vi "Update UI Captions.vi"(7 "Diagnostic Protocol":T1, 8 "error in (no error)":errorcluster, 10 "Cmd":T3, 11 "UI.Refs":T2) -> (0 "error out":errorcluster)   [LabVIEW 2015, in "Diagnostics Addon Shared.lvlib"]
uses:
  Diagnostics Addon Shared.lvlib
  Types/Channel Commands Enum.ctl
  Types/UI.Refs.ctl
  Types/Diagnostic Protocols.ctl
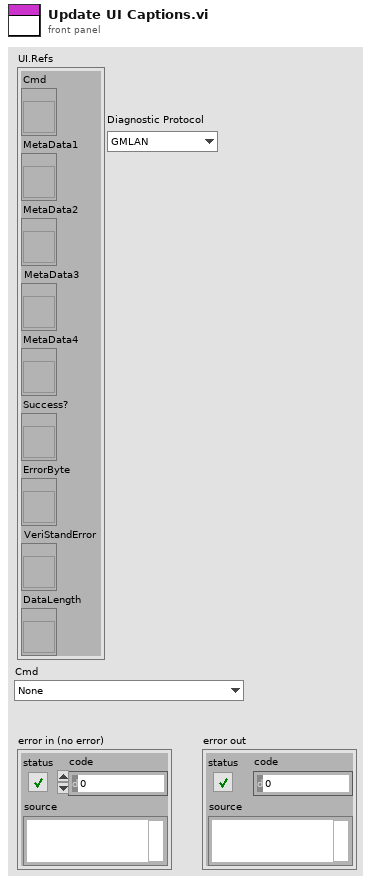
[diagram p1: front panel]
types:
  T1 = typedef "Diagnostics Addon Shared.lvlib/Diagnostic Protocols.ctl" = enum16{"GMLAN", "KWP-2000", "UDS"}
  T2 = typedef "Diagnostics Addon Shared.lvlib/UI.Refs.ctl" = cluster{"Cmd":refnum<vi>, "MetaData1":refnum<vi>, "MetaData2":refnum<vi>, "MetaData3":refnum<vi>, "MetaData4":refnum<vi>, "Success?":refnum<vi>, "ErrorByte":refnum<vi>, "VeriStandError":refnum<vi>, "DataLength":refnum<vi>}
  T3 = typedef "Diagnostics Addon Shared.lvlib/Channel Commands Enum.ctl" = enum8{"None", "EnableDiagnosticSession", "DisableDiagnosticSession", "ReadDataIdentifiers", "ReadDataIdentifier", "WriteDataIndentifier", "ReadPIDsOnDemand", "ReadPIDOnDemand", "WriteCPID", "WriteMemory", "ReadMemory", "ReadDTCs", "ClearDTCs", "ControlDTC", "ForceTesterPresent", "DisableNormalCommunication", "ReturnToNormalMode", "InputOutputControl", "StartRoutine", "RequestRoutineStatus", "StopRoutine", "ECUReset", "UnlockECU", "ClearSuccessBit", "ConfigureandStartPIDs", "StopPIDs", "StartDTCs", "EnableChangeDTCCount", "DisableChangeDTCCount", "ReadFailureRecordParameters", "PassThru Channel Based"}
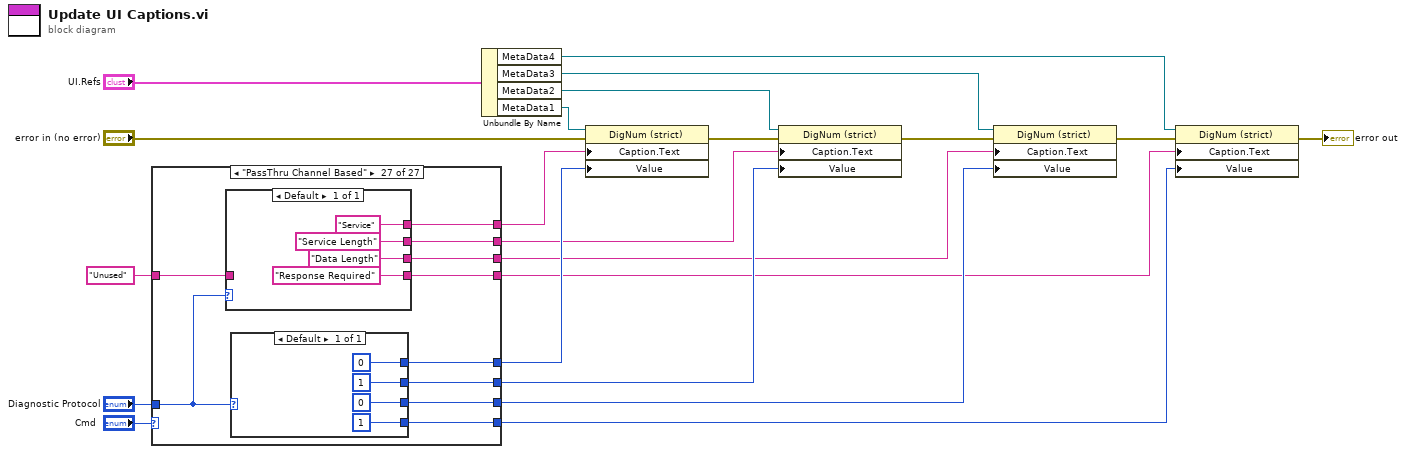
[diagram p0: block diagram]
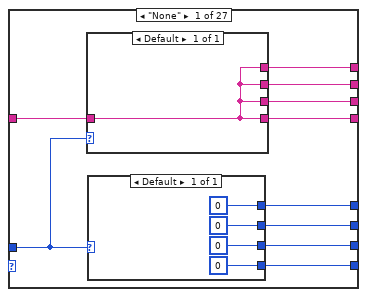
[diagram p2: hidden frame]
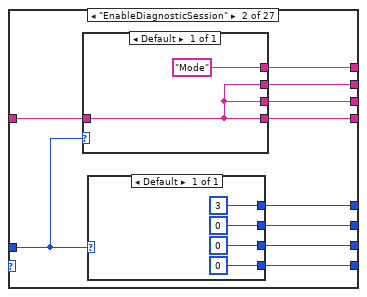
[diagram p3: hidden frame]
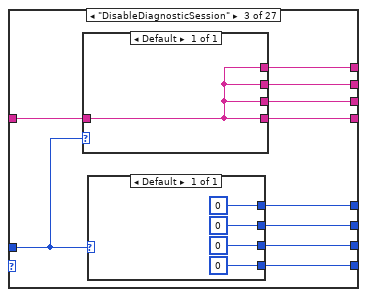
[diagram p4: hidden frame]
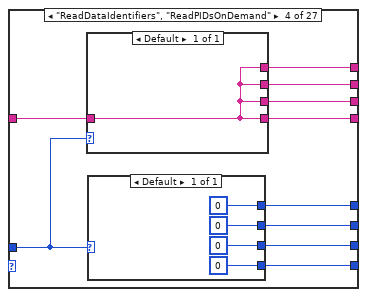
[diagram p5: hidden frame]
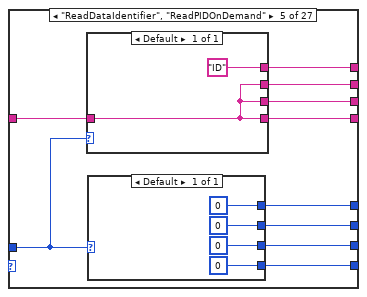
[diagram p6: hidden frame]
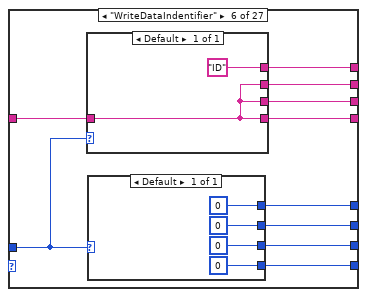
[diagram p7: hidden frame]
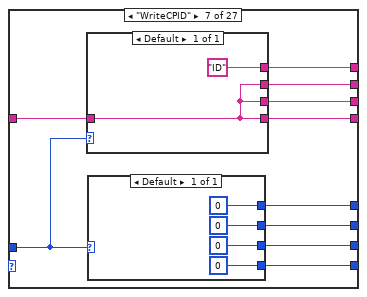
[diagram p8: hidden frame]
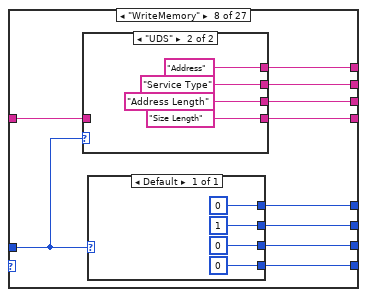
[diagram p9: hidden frame]
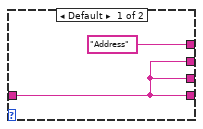
[diagram p10: hidden frame]
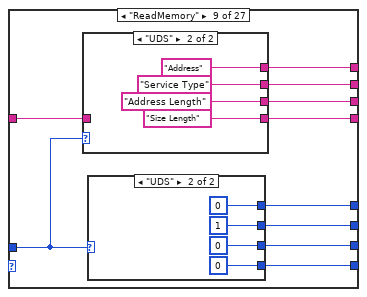
[diagram p11: hidden frame]
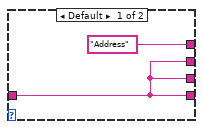
[diagram p12: hidden frame]
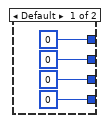
[diagram p13: hidden frame]
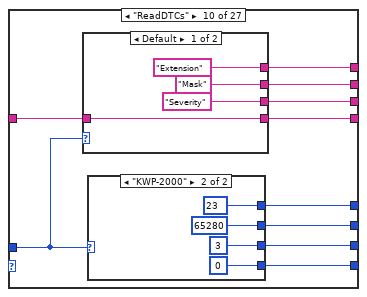
[diagram p14: hidden frame]
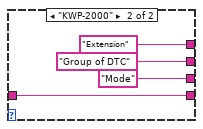
[diagram p15: hidden frame]
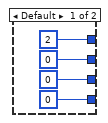
[diagram p16: hidden frame]
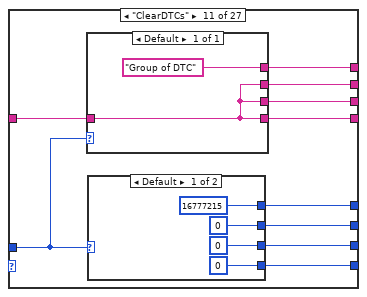
[diagram p17: hidden frame]
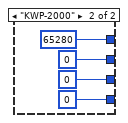
[diagram p18: hidden frame]
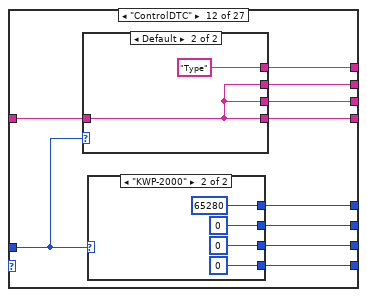
[diagram p19: hidden frame]
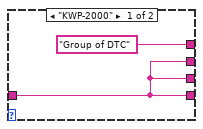
[diagram p20: hidden frame]
diagram:
  n1 = case shown="\"PassThru Channel Based\"" "Cmd" {
    tunnel: [w27 w42 w58 w73 w88 w104 w120 w136 w156 w180 w206 w226 w248 w264 w281 w296 w317 w333 w349 w364 w379 w394 w409 w425 w441 w457 w475] -> w20
    tunnel: [w31 w46 w62 w77 w92 w108 w124 w140 w160 w184 w210 w230 w252 w268 w285 w300 w321 w337 w353 w368 w383 w398 w413 w429 w445 w461 w479] -> w21
    tunnel: [w25 w40 w56 w71 w86 w102 w118 w134 w154 w178 w204 w224 w246 w262 w279 w294 w315 w331 w347 w362 w377 w392 w407 w423 w439 w455 w473] -> w8
    tunnel: [w30 w45 w61 w76 w91 w107 w123 w139 w159 w183 w209 w229 w251 w267 w284 w299 w320 w336 w352 w367 w382 w397 w412 w428 w444 w460 w478] -> w7
    tunnel: [w23 w38 w54 w69 w84 w100 w116 w132 w152 w176 w202 w222 w244 w260 w277 w292 w313 w329 w345 w360 w375 w390 w405 w421 w437 w453 w471] -> w6
    tunnel: [w29 w44 w60 w75 w90 w106 w122 w138 w158 w182 w208 w228 w250 w266 w283 w298 w319 w335 w351 w366 w381 w396 w411 w427 w443 w459 w477] -> w5
    tunnel: [w22 w37 w53 w68 w83 w99 w115 w131 w151 w175 w201 w221 w243 w259 w276 w291 w312 w328 w344 w359 w374 w389 w404 w420 w436 w452 w470] -> w4
    tunnel: [w28 w43 w59 w74 w89 w105 w121 w137 w157 w181 w207 w227 w249 w265 w282 w297 w318 w334 w350 w365 w380 w395 w410 w426 w442 w458 w476] -> w3
    tunnel: "Unused" -> [w24 w39 w55 w70 w85 w101 w117 w133 w153 w177 w203 w223 w245 w261 w278 w293 w314 w330 w346 w361 w376 w391 w406 w422 w438 w454 w472]
    tunnel: "Diagnostic Protocol" -> [w26 w41 w57 w72 w87 w103 w119 w135 w155 w179 w205 w225 w247 w263 w280 w295 w316 w332 w348 w363 w378 w393 w408 w424 w440 w456 w474]
    frame "None" {
      n2 = case shown="Default" w26 {
        tunnel: [w32] -> w27
        tunnel: [w32] -> w25
        tunnel: w24 -> [w32]
        tunnel: [w32] -> w23
        tunnel: [w32] -> w22
        frame Default {
        }
      }
      n3 = case shown="Default" w26 {
        tunnel: [i64 0 ("Value")] -> w31
        tunnel: [i64 0 ("Value")] -> w30
        tunnel: [i64 0 ("Value")] -> w29
        tunnel: [i64 0 ("Value")] -> w28
        frame Default {
        }
      }
    }
    frame "EnableDiagnosticSession" {
      n4 = case shown="Default" w41 {
        tunnel: ["Mode"] -> w42
        tunnel: [w48] -> w40
        tunnel: w39 -> [w48]
        tunnel: [w48] -> w38
        tunnel: [w48] -> w37
        frame Default {
        }
      }
      n5 = case shown="Default" w41 {
        tunnel: [i64 3 ("Value")] -> w46
        tunnel: [i64 0 ("Value")] -> w45
        tunnel: [i64 0 ("Value")] -> w44
        tunnel: [i64 0 ("Value")] -> w43
        frame Default {
        }
      }
    }
    frame "DisableDiagnosticSession" {
      n6 = case shown="Default" w57 {
        tunnel: [w63] -> w58
        tunnel: [w63] -> w56
        tunnel: w55 -> [w63]
        tunnel: [w63] -> w54
        tunnel: [w63] -> w53
        frame Default {
        }
      }
      n7 = case shown="Default" w57 {
        tunnel: [i64 0 ("Value")] -> w62
        tunnel: [i64 0 ("Value")] -> w61
        tunnel: [i64 0 ("Value")] -> w60
        tunnel: [i64 0 ("Value")] -> w59
        frame Default {
        }
      }
    }
    frame "ReadDataIdentifiers", "ReadPIDsOnDemand" {
      n8 = case shown="Default" w72 {
        tunnel: [w78] -> w73
        tunnel: [w78] -> w71
        tunnel: w70 -> [w78]
        tunnel: [w78] -> w69
        tunnel: [w78] -> w68
        frame Default {
        }
      }
      n9 = case shown="Default" w72 {
        tunnel: [i64 0 ("Value")] -> w77
        tunnel: [i64 0 ("Value")] -> w76
        tunnel: [i64 0 ("Value")] -> w75
        tunnel: [i64 0 ("Value")] -> w74
        frame Default {
        }
      }
    }
    frame "ReadDataIdentifier", "ReadPIDOnDemand" {
      n10 = case shown="Default" w87 {
        tunnel: ["ID"] -> w88
        tunnel: [w94] -> w86
        tunnel: w85 -> [w94]
        tunnel: [w94] -> w84
        tunnel: [w94] -> w83
        frame Default {
        }
      }
      n11 = case shown="Default" w87 {
        tunnel: [i64 0 ("Value")] -> w92
        tunnel: [i64 0 ("Value")] -> w91
        tunnel: [i64 0 ("Value")] -> w90
        tunnel: [i64 0 ("Value")] -> w89
        frame Default {
        }
      }
    }
    frame "WriteDataIndentifier" {
      n12 = case shown="Default" w103 {
        tunnel: ["ID"] -> w104
        tunnel: [w110] -> w102
        tunnel: w101 -> [w110]
        tunnel: [w110] -> w100
        tunnel: [w110] -> w99
        frame Default {
        }
      }
      n13 = case shown="Default" w103 {
        tunnel: [i64 0 ("Value")] -> w108
        tunnel: [i64 0 ("Value")] -> w107
        tunnel: [i64 0 ("Value")] -> w106
        tunnel: [i64 0 ("Value")] -> w105
        frame Default {
        }
      }
    }
    frame "WriteCPID" {
      n14 = case shown="Default" w119 {
        tunnel: ["ID"] -> w120
        tunnel: [w126] -> w118
        tunnel: w117 -> [w126]
        tunnel: [w126] -> w116
        tunnel: [w126] -> w115
        frame Default {
        }
      }
      n15 = case shown="Default" w119 {
        tunnel: [i64 0 ("Value")] -> w124
        tunnel: [i64 0 ("Value")] -> w123
        tunnel: [i64 0 ("Value")] -> w122
        tunnel: [i64 0 ("Value")] -> w121
        frame Default {
        }
      }
    }
    frame "WriteMemory" {
      n16 = case shown="\"UDS\"" w135 {
        tunnel: ["Address" "Address"] -> w136
        tunnel: [w141 "Service Type"] -> w134
        tunnel: w133 -> [w141 _]
        tunnel: [w141 "Address Length"] -> w132
        tunnel: [w141 "Size Length"] -> w131
        frame Default {
        }
        frame "UDS" {
        }
      }
      n17 = case shown="Default" w135 {
        tunnel: [i64 0 ("Value")] -> w140
        tunnel: [i64 1 ("Value")] -> w139
        tunnel: [i64 0 ("Value")] -> w138
        tunnel: [i64 0 ("Value")] -> w137
        frame Default {
        }
      }
    }
    frame "ReadMemory" {
      n18 = case shown="\"UDS\"" w155 {
        tunnel: ["Address" "Address"] -> w156
        tunnel: [w161 "Service Type"] -> w154
        tunnel: w153 -> [w161 _]
        tunnel: [w161 "Address Length"] -> w152
        tunnel: [w161 "Size Length"] -> w151
        frame Default {
        }
        frame "UDS" {
        }
      }
      n19 = case shown="\"UDS\"" w155 {
        tunnel: [i64 0 ("Value") i64 0 ("Value")] -> w160
        tunnel: [i64 0 ("Value") i64 1 ("Value")] -> w159
        tunnel: [i64 0 ("Value") i64 0 ("Value")] -> w158
        tunnel: [i64 0 ("Value") i64 0 ("Value")] -> w157
        frame Default {
        }
        frame "UDS" {
        }
      }
    }
    frame "ReadDTCs" {
      n20 = case shown="Default" w179 {
        tunnel: ["Extension" "Extension"] -> w180
        tunnel: ["Mask" "Group of DTC"] -> w178
        tunnel: w177 -> [w187 w191]
        tunnel: ["Severity" "Mode"] -> w176
        tunnel: [w187 w191] -> w175
        frame Default {
        }
        frame "KWP-2000" {
        }
      }
      n21 = case shown="\"KWP-2000\"" w179 {
        tunnel: [i64 2 ("Value") i64 23 ("Value")] -> w184
        tunnel: [i64 0 ("Value") i64 65280 ("Value")] -> w183
        tunnel: [i64 0 ("Value") i64 3 ("Value")] -> w182
        tunnel: [i64 0 ("Value") i64 0 ("Value")] -> w181
        frame Default {
        }
        frame "KWP-2000" {
        }
      }
    }
    frame "ClearDTCs" {
      n22 = case shown="Default" w205 {
        tunnel: ["Group of DTC"] -> w206
        tunnel: [w211] -> w204
        tunnel: w203 -> [w211]
        tunnel: [w211] -> w202
        tunnel: [w211] -> w201
        frame Default {
        }
      }
      n23 = case shown="Default" w205 {
        tunnel: [i64 16777215 ("Value") i64 65280 ("Value")] -> w210
        tunnel: [i64 0 ("Value") i64 0 ("Value")] -> w209
        tunnel: [i64 0 ("Value") i64 0 ("Value")] -> w208
        tunnel: [i64 0 ("Value") i64 0 ("Value")] -> w207
        frame Default {
        }
        frame "KWP-2000" {
        }
      }
    }
    frame "ControlDTC" {
      n24 = case shown="Default" w225 {
        tunnel: ["Group of DTC" "Type"] -> w226
        tunnel: [w231 w233] -> w224
        tunnel: w223 -> [w231 w233]
        tunnel: [w231 w233] -> w222
        tunnel: [w231 w233] -> w221
        frame "KWP-2000" {
        }
        frame Default {
        }
      }
      n25 = case shown="\"KWP-2000\"" w225 {
        tunnel: [i64 1 ("Value") i64 65280 ("Value")] -> w230
        tunnel: [i64 0 ("Value") i64 0 ("Value")] -> w229
        tunnel: [i64 0 ("Value") i64 0 ("Value")] -> w228
        tunnel: [i64 0 ("Value") i64 0 ("Value")] -> w227
        frame Default {
        }
        frame "KWP-2000" {
        }
      }
    }
    frame "ForceTesterPresent" {
      n26 = case shown="Default" w247 {
        tunnel: ["Require Response?"] -> w248
        tunnel: [w253] -> w246
        tunnel: w245 -> [w253]
        tunnel: [w253] -> w244
        tunnel: [w253] -> w243
        frame Default {
        }
      }
      n27 = case shown="Default" w247 {
        tunnel: [i64 1 ("Value")] -> w252
        tunnel: [i64 0 ("Value")] -> w251
        tunnel: [i64 0 ("Value")] -> w250
        tunnel: [i64 0 ("Value")] -> w249
        frame Default {
        }
      }
    }
    frame "DisableNormalCommunication" {
      n28 = case shown="Default" w263 {
        tunnel: ["Type"] -> w264
        tunnel: ["Comm Type"] -> w262
        tunnel: w261 -> [w270]
        tunnel: [w270] -> w260
        tunnel: [w270] -> w259
        frame Default {
        }
      }
      n29 = case shown="Default" w263 {
        tunnel: [i64 1 ("Value")] -> w268
        tunnel: [i64 3 ("Value")] -> w267
        tunnel: [i64 0 ("Value")] -> w266
        tunnel: [i64 0 ("Value")] -> w265
        frame Default {
        }
      }
    }
    frame "ReturnToNormalMode" {
      n30 = case shown="Default" w280 {
        tunnel: [w286] -> w281
        tunnel: [w286] -> w279
        tunnel: w278 -> [w286]
        tunnel: [w286] -> w277
        tunnel: [w286] -> w276
        frame Default {
        }
      }
      n31 = case shown="Default" w280 {
        tunnel: [i64 0 ("Value")] -> w285
        tunnel: [i64 0 ("Value")] -> w284
        tunnel: [i64 0 ("Value")] -> w283
        tunnel: [i64 0 ("Value")] -> w282
        frame Default {
        }
      }
    }
    frame "InputOutputControl" {
      n32 = case shown="Default" w295 {
        tunnel: ["ID"] -> w296
        tunnel: ["Mode"] -> w294
        tunnel: w293 -> [w303]
        tunnel: [w303] -> w292
        tunnel: [w303] -> w291
        frame Default {
        }
      }
      n33 = case shown="Default" w295 {
        tunnel: [i64 0 ("Value") i64 0 ("Value")] -> w300
        tunnel: [i64 3 ("Value") i64 7 ("Value")] -> w299
        tunnel: [i64 0 ("Value") i64 0 ("Value")] -> w298
        tunnel: [i64 0 ("Value") i64 0 ("Value")] -> w297
        frame Default {
        }
        frame "KWP-2000" {
        }
      }
    }
    frame "StartRoutine".."StopRoutine" {
      n34 = case shown="Default" w316 {
        tunnel: ["ID"] -> w317
        tunnel: [w322] -> w315
        tunnel: w314 -> [w322]
        tunnel: [w322] -> w313
        tunnel: [w322] -> w312
        frame Default {
        }
      }
      n35 = case shown="Default" w316 {
        tunnel: [i64 0 ("Value")] -> w321
        tunnel: [i64 0 ("Value")] -> w320
        tunnel: [i64 0 ("Value")] -> w319
        tunnel: [i64 0 ("Value")] -> w318
        frame Default {
        }
      }
    }
    frame "ECUReset" {
      n36 = case shown="Default" w332 {
        tunnel: ["Mode"] -> w333
        tunnel: [w338] -> w331
        tunnel: w330 -> [w338]
        tunnel: [w338] -> w329
        tunnel: [w338] -> w328
        frame Default {
        }
      }
      n37 = case shown="Default" w332 {
        tunnel: [i64 1 ("Value")] -> w337
        tunnel: [i64 0 ("Value")] -> w336
        tunnel: [i64 0 ("Value")] -> w335
        tunnel: [i64 0 ("Value")] -> w334
        frame Default {
        }
      }
    }
    frame "UnlockECU" {
      n38 = case shown="Default" w348 {
        tunnel: [w354] -> w349
        tunnel: [w354] -> w347
        tunnel: w346 -> [w354]
        tunnel: [w354] -> w345
        tunnel: [w354] -> w344
        frame Default {
        }
      }
      n39 = case shown="Default" w348 {
        tunnel: [i64 0 ("Value")] -> w353
        tunnel: [i64 0 ("Value")] -> w352
        tunnel: [i64 0 ("Value")] -> w351
        tunnel: [i64 0 ("Value")] -> w350
        frame Default {
        }
      }
    }
    frame "ClearSuccessBit" {
      n40 = case shown="Default" w363 {
        tunnel: [w369] -> w364
        tunnel: [w369] -> w362
        tunnel: w361 -> [w369]
        tunnel: [w369] -> w360
        tunnel: [w369] -> w359
        frame Default {
        }
      }
      n41 = case shown="Default" w363 {
        tunnel: [i64 0 ("Value")] -> w368
        tunnel: [i64 0 ("Value")] -> w367
        tunnel: [i64 0 ("Value")] -> w366
        tunnel: [i64 0 ("Value")] -> w365
        frame Default {
        }
      }
    }
    frame "ConfigureandStartPIDs" {
      n42 = case shown="Default" w378 {
        tunnel: [w384] -> w379
        tunnel: [w384] -> w377
        tunnel: w376 -> [w384]
        tunnel: [w384] -> w375
        tunnel: [w384] -> w374
        frame Default {
        }
      }
      n43 = case shown="Default" w378 {
        tunnel: [i64 0 ("Value")] -> w383
        tunnel: [i64 0 ("Value")] -> w382
        tunnel: [i64 0 ("Value")] -> w381
        tunnel: [i64 0 ("Value")] -> w380
        frame Default {
        }
      }
    }
    frame "StopPIDs" {
      n44 = case shown="Default" w393 {
        tunnel: [w399] -> w394
        tunnel: [w399] -> w392
        tunnel: w391 -> [w399]
        tunnel: [w399] -> w390
        tunnel: [w399] -> w389
        frame Default {
        }
      }
      n45 = case shown="Default" w393 {
        tunnel: [i64 0 ("Value")] -> w398
        tunnel: [i64 0 ("Value")] -> w397
        tunnel: [i64 0 ("Value")] -> w396
        tunnel: [i64 0 ("Value")] -> w395
        frame Default {
        }
      }
    }
    frame "StartDTCs" {
      n46 = case shown="Default" w408 {
        tunnel: ["Status Mask"] -> w409
        tunnel: [w414] -> w407
        tunnel: w406 -> [w414]
        tunnel: [w414] -> w405
        tunnel: [w414] -> w404
        frame Default {
        }
      }
      n47 = case shown="Default" w408 {
        tunnel: [i64 2 ("Value")] -> w413
        tunnel: [i64 0 ("Value")] -> w412
        tunnel: [i64 0 ("Value")] -> w411
        tunnel: [i64 0 ("Value")] -> w410
        frame Default {
        }
      }
    }
    frame "EnableChangeDTCCount" {
      n48 = case shown="Default" w424 {
        tunnel: ["Status Mask"] -> w425
        tunnel: [w430] -> w423
        tunnel: w422 -> [w430]
        tunnel: [w430] -> w421
        tunnel: [w430] -> w420
        frame Default {
        }
      }
      n49 = case shown="Default" w424 {
        tunnel: [i64 2 ("Value")] -> w429
        tunnel: [i64 0 ("Value")] -> w428
        tunnel: [i64 0 ("Value")] -> w427
        tunnel: [i64 0 ("Value")] -> w426
        frame Default {
        }
      }
    }
    frame "DisableChangeDTCCount" {
      n50 = case shown="Default" w440 {
        tunnel: ["Status Mask"] -> w441
        tunnel: [w446] -> w439
        tunnel: w438 -> [w446]
        tunnel: [w446] -> w437
        tunnel: [w446] -> w436
        frame Default {
        }
      }
      n51 = case shown="Default" w440 {
        tunnel: [i64 0 ("Value")] -> w445
        tunnel: [i64 0 ("Value")] -> w444
        tunnel: [i64 0 ("Value")] -> w443
        tunnel: [i64 0 ("Value")] -> w442
        frame Default {
        }
      }
    }
    frame "ReadFailureRecordParameters" {
      n52 = case shown="Default" w456 {
        tunnel: ["ID"] -> w457
        tunnel: ["Failure Type"] -> w455
        tunnel: w454 -> [w465]
        tunnel: ["Failure Record Number"] -> w453
        tunnel: [w465] -> w452
        frame Default {
        }
      }
      n53 = case shown="Default" w456 {
        tunnel: [i64 0 ("Value")] -> w461
        tunnel: [i64 0 ("Value")] -> w460
        tunnel: [i64 0 ("Value")] -> w459
        tunnel: [i64 0 ("Value")] -> w458
        frame Default {
        }
      }
    }
    frame "PassThru Channel Based" {
      n54 = case shown="Default" w474 {
        tunnel: ["Service"] -> w475
        tunnel: ["Service Length"] -> w473
        tunnel: w472 -> [_]
        tunnel: ["Data Length"] -> w471
        tunnel: ["Response Required"] -> w470
        frame Default {
        }
      }
      n55 = case shown="Default" w474 {
        tunnel: [i64 0 ("Value")] -> w479
        tunnel: [i64 1 ("Value")] -> w478
        tunnel: [i64 0 ("Value")] -> w477
        tunnel: [i64 1 ("Value")] -> w476
        frame Default {
        }
      }
    }
  }
  n56 = Unbundle By Name("UI.Refs") -> ("MetaData4"=w9:refnum<vi>, "MetaData3"=w10:refnum<vi>, "MetaData2"=w11:refnum<vi>, "MetaData1"=w18:refnum<vi>)
  n57 = property class="DigNum (strict)"(reference=w18, error in="error in (no error)", "Caption.Text"=w20, "Value"=w21) -> (error out=w15:errorcluster)  [unwired: 1 out]
  n58 = property class="DigNum (strict)"(reference=w11, error in=w15, "Caption.Text"=w8, "Value"=w7) -> (error out=w14:errorcluster)  [unwired: 1 out]
  n59 = property class="DigNum (strict)"(reference=w10, error in=w14, "Caption.Text"=w6, "Value"=w5) -> (error out=w13:errorcluster)  [unwired: 1 out]
  n60 = property class="DigNum (strict)"(reference=w9, error in=w13, "Caption.Text"=w4, "Value"=w3) -> (error out=→"error out":errorcluster)  [unwired: 1 out]
